vi "Parse ITX String.vi"(8 "error in (no error)":errorcluster, 11 "ITX String":string) -> (0 "error out":errorcluster, 1 "Commands":string, 2 "Notes":string, 3 "Data (Dictionary)":T1[](array[typedef]))   [LabVIEW 2019, in "LV-Data.ITX.lvclass"]
uses:
  LV-Data.ITX.lvclass
  LV-Data/Typedefs/Dictionary--cluster.ctl
  <userlib>/_OpenG.lib/string/string.llb/Trim Whitespace (String)__ogtk.vi
  LV-Data/LV-Data.lvclass
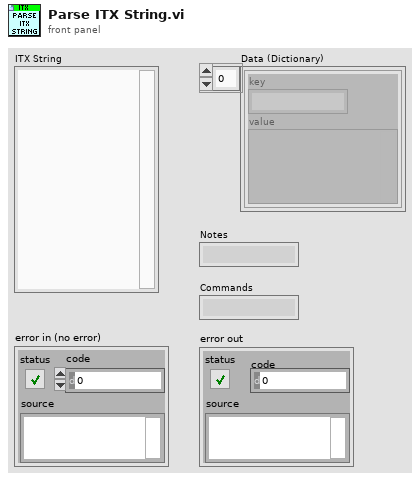
[diagram p1: front panel]
types:
  T1 = typedef "LV-Data.lvclass/Dictionary--cluster.ctl" = cluster{"key":string, "value":variant}
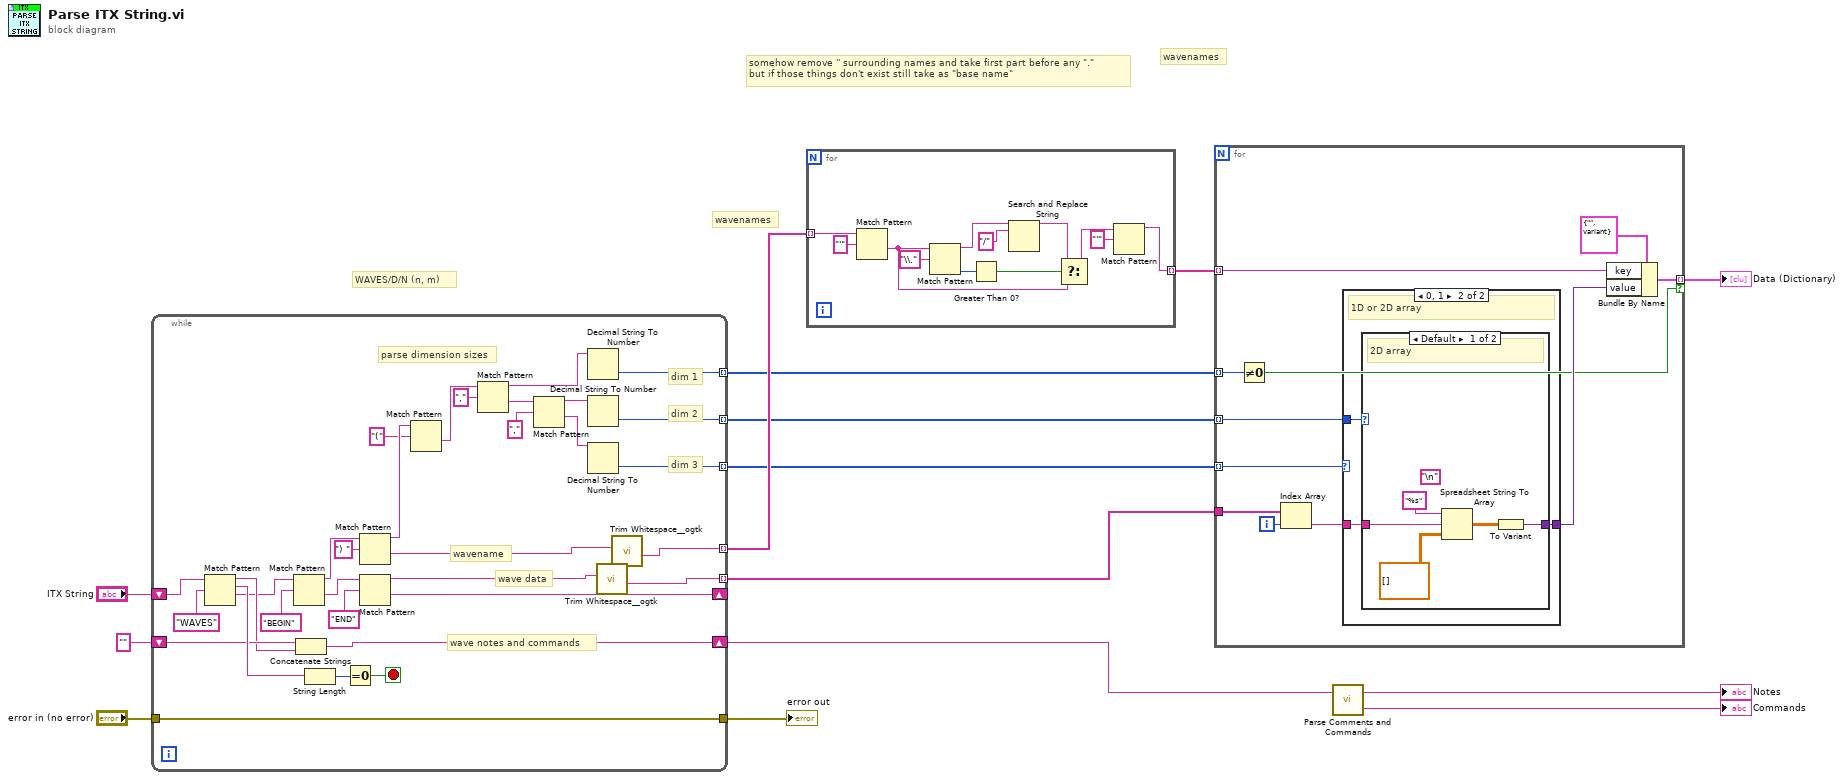
[diagram p0: block diagram]
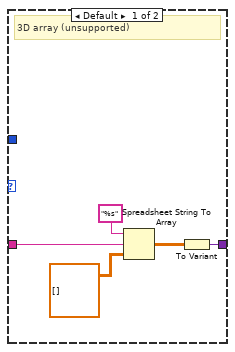
[diagram p2: hidden frame]
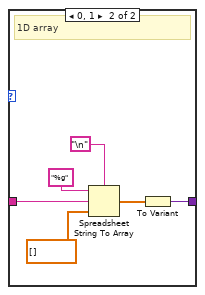
[diagram p3: hidden frame]
diagram:
  # "wavenames"
  # "wavenames"
  # "somehow remove '' surrounding names and take first part before any \".\"\nbut if those things don't exist still take as \"base name\""
  # "WAVES/D/N (n, m)"
  n1 = while {
    tunnel: [w22] -> w10 mode=indexing
    shift-right: [w45] -> _
    shift-left: "ITX String" -> [w34]
    tunnel: [w15] -> w8 mode=indexing
    shift-right: [w37] -> w1
    shift-left: "" ("regular expression") -> [w36]
    tunnel: [w32] -> w11
    tunnel: "error in (no error)" -> [w32]
    tunnel: [w24] -> w5 mode=indexing
    tunnel: [w26] -> w6 mode=indexing
    tunnel: [w17] -> w7 mode=indexing
    stop <- w42 stop-if-true
    # "dim 3"
    # "dim 2"
    # "dim 1"
    # "wave data"
    # "wave notes and commands"
    # "parse dimension sizes"
    # "wavename"
    n2 = Match Pattern(string=w34, regular expression="WAVES") -> (before substring=w35:string, match substring=w44:string, after substring=w31:string)  [unwired: 2 out]
    n3 = Match Pattern(string=w31, regular expression="BEGIN" ("regular expression 2")) -> (before substring=w33:string, after substring=w46:string)  [unwired: 3 out]
    n4 = Concatenate Strings(w36, w35) -> (w37:string)
    n5 = String Length(string=w44) -> (length=w43:i32)
    n6 = Equal To 0?(x=w43) -> (x = 0?=w42:bool)
    n7 = Match Pattern(string=w33, regular expression=") ") -> (before substring=w30:string, after substring=w16:string)  [unwired: 3 out]
    n8 = Match Pattern(string=w46, regular expression="END" ("regular expression 3")) -> (before substring=w23:string, after substring=w45:string)  [unwired: 3 out]
    n9 = Match Pattern(string=w30, regular expression="(") -> (after substring=w28:string)  [unwired: 4 out]
    n10 = Match Pattern(string=w28, regular expression=",") -> (before substring=w25:string, after substring=w21:string)  [unwired: 3 out]
    n11 = Match Pattern(string=w21, regular expression=",") -> (before substring=w19:string, after substring=w20:string)  [unwired: 3 out]
    n12 = Decimal String To Number(string=w25) -> (number=w24:i32)  [unwired: 2 in, 1 out]
    n13 = Decimal String To Number(string=w19) -> (number=w26:i32)  [unwired: 2 in, 1 out]
    n14 = Decimal String To Number(string=w20) -> (number=w17:i32)  [unwired: 2 in, 1 out]
    n15 = call-poly <userlib>:"Trim Whitespace__ogtk.vi"("String in"=w23) -> ("String out"=w22:string)  [unwired: 6 in]
    n16 = call-poly <userlib>:"Trim Whitespace__ogtk.vi"("String in"=w16) -> ("String out"=w15:string)  [unwired: 6 in]
  }
  "error out" <- w11
  n17 = for {
    tunnel: w8 -> [w48] mode=indexing
    tunnel: [w50] -> w9 mode=indexing
    n18 = Match Pattern(string=w48, regular expression="'") -> (after substring=w49:string)  [unwired: 4 out]
    n19 = Match Pattern(string=w49, regular expression="\\.") -> (before substring=w55:string, offset past match=w57:i32)  [unwired: 1 in, 2 out]
    n20 = Greater Than 0?(x=w57) -> (x > 0?=w54:bool)
    n21 = Search and Replace String(input string=w55, search string="/") -> (result string=w53:string)  [unwired: 6 in, 3 out]
    n22 = Select(t=w53, s=w54, f=w49) -> (s? t:f=w47:string)
    n23 = Match Pattern(string=w47, regular expression="'") -> (before substring=w50:string)  [unwired: 4 out]
  }
  n24 = for {
    tunnel: w10 -> [w69]
    tunnel: w9 -> [w62] mode=indexing
    tunnel: [w67] -> w12 mode=indexing if=w59
    tunnel: w5 -> [w60] mode=indexing
    tunnel: w6 -> [w64] mode=indexing
    tunnel: w7 -> [w65] mode=indexing
    i -> [w68]
    n25 = Not Equal To 0?(x=w60) -> (x != 0?=w59:bool)
    n26 = Index Array(array=w69, index=w68) -> (element=w63:string)
    n27 = case shown="0, 1" w65 {
      tunnel: w63 -> [w72 w76]
      tunnel: [w74 w77] -> w61
      tunnel: w64 -> [_ w75]
      frame Default {
        # "3D array (unsupported)"
        n28 = Spreadsheet String To Array(format string="%s", spreadsheet string=w72, array type (2D Dbl)=dbl[][][] []) -> (array=w71:dbl[][][])  [unwired: 1 out]
        n29 = To Variant(anything=w71) -> (Variant=w74:variant)
      }
      frame 0, 1 {
        # "1D or 2D array"
        n30 = case shown="Default" w75 {
          tunnel: [w82 w88] -> w77
          tunnel: w76 -> [w80 w87]
          frame Default {
            (unwired) "\n"
            # "2D array"
            n31 = Spreadsheet String To Array(format string="%s", spreadsheet string=w80, array type (2D Dbl)=dbl[][] []) -> (array=w79:dbl[][])  [unwired: 1 out]
            n32 = To Variant(anything=w79) -> (Variant=w82:variant)
          }
          frame 0, 1 {
            # "1D array"
            n33 = Spreadsheet String To Array(delimiter (Tab)="\n", format string="%g", spreadsheet string=w87, array type (2D Dbl)=dbl[] []) -> (array=w86:dbl[])
            n34 = To Variant(anything=w86) -> (Variant=w88:variant)
          }
        }
      }
    }
    n35 = Bundle By Name(cluster=T1 {"key"="", "value"=variant} ("key-value"), "key"=w62, "value"=w61) -> (w67:T1)
  }
  "Data (Dictionary)" <- w12
  n36 = call "Parse Comments and Commands.vi"("ITX Notes and Commands"=w1) -> ("Commands"=→"Commands":string, "Notes"=→"Notes":string)  [unwired: 1 in]
